vi "Get Items.vi"(8 "error in (no error)":errorcluster caption="错误输入（无错误）", 11 "Section输入":refnum<class "Section.lvclass">) -> (0 "error out":errorcluster caption="错误输出", 2 "Items":refnum<data-value>[](array[refnum]), 3 "Section输出":refnum<class "Section.lvclass">)   [LabVIEW 2013, in "Hierarchy Framework.lvlib" / "Section.lvclass"]
uses:
  Section.lvclass
  Item/Item.lvclass
  Section.lvclass/Section.ctl
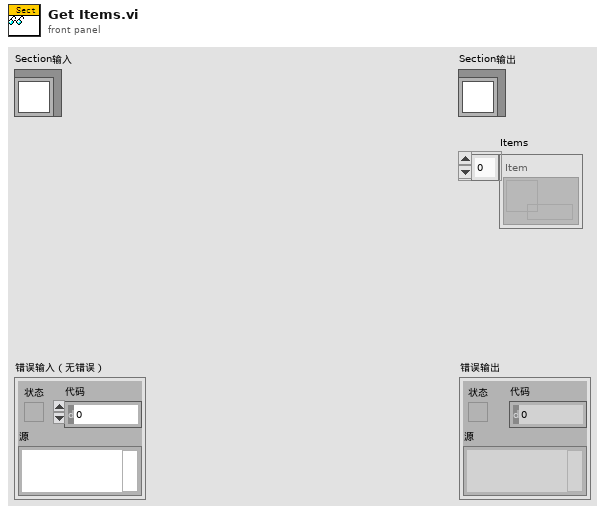
[diagram p1: front panel]
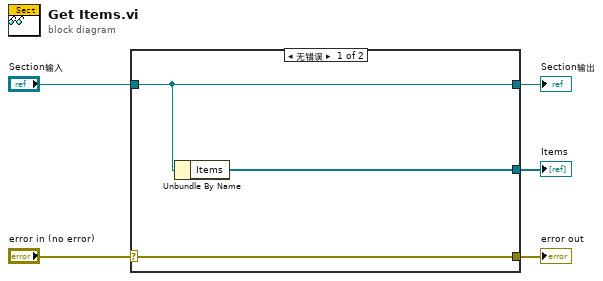
[diagram p0: block diagram]
diagram:
  n1 = case shown="无错误" "error in (no error)" {
    selector: "error in (no error)" -> [w8 w9]
    tunnel: [w8 w9] -> w4
    tunnel: [w7 w10] -> w2
    tunnel: "Section输入" -> [w7 w10]
    tunnel: [w6 _] -> w1
    frame No Error {
      n2 = Unbundle By Name(w7) -> ("Items"=w6:refnum<data-value>[])
    }
    frame Error {
    }
  }
  "error out" <- w4
  "Section输出" <- w2
  "Items" <- w1
